vi "Update State Description.vi"(8 "error in (no error)":errorcluster, 9 "description":string, 10 "State":string, 11 "Channel Ref in":T1 format="%.0x") -> (0 "error out":errorcluster, 3 "Channel Ref out":T1=18446744073709551615 format="%.0x")   [LabVIEW 2017, in "Switch Scripting.lvlib"]
uses:
  Switch Scripting.lvlib
  <vilib>/NI Veristand/Custom Device API/Custom Device Item Ref.ctl
  <vilib>/NI VeriStand/Custom Device API/Custom Device API.lvlib
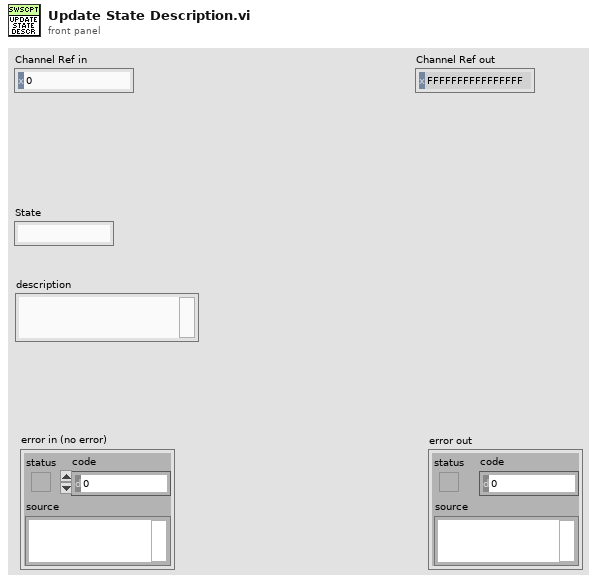
[diagram p1: front panel]
types:
  T1 = typedef "Custom Device API.lvlib/Custom Device Item Ref.ctl" = u64
  T2 = typedef "Switch Scripting.lvlib/Routing State.ctl" = cluster{"name":string, "description":string, "value":i32, "connection list":T3[]}
  T3 = typedef "Switch Scripting.lvlib/Connection.ctl" = cluster{"source":string, "destination":string}
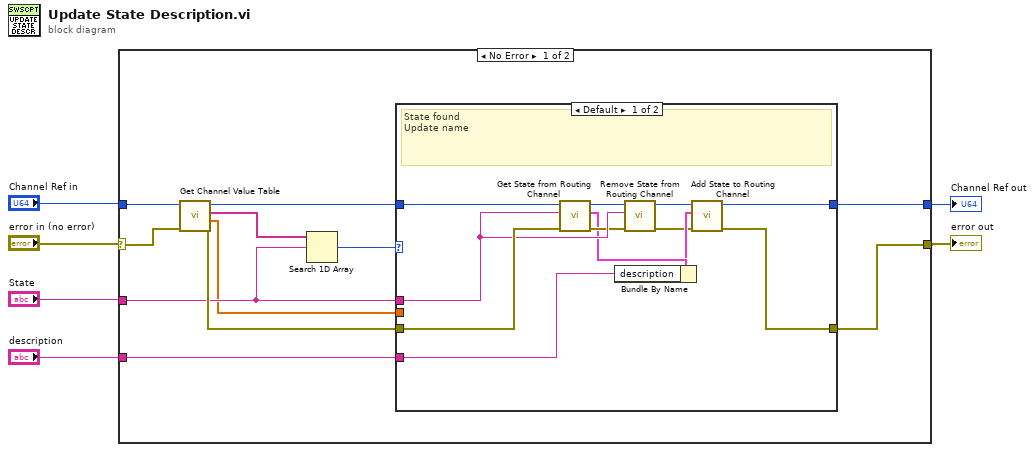
[diagram p0: block diagram]
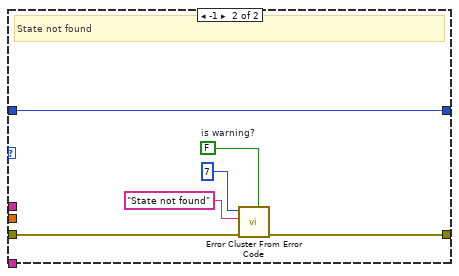
[diagram p2: hidden frame]
diagram:
  n1 = case shown="No Error" "error in (no error)" {
    selector: "error in (no error)" -> [w16 w37]
    tunnel: [w12 w37] -> w2
    tunnel: "Channel Ref in" -> [w17 w36]
    tunnel: [w13 w36] -> w1
    tunnel: "State" -> [w10 _]
    tunnel: "description" -> [w8 _]
    frame No Error {
      n2 = call "Get Channel Value Table.vi"("error in (no error)"=w16, "Channel Ref in"=w17) -> ("error out"=w14:errorcluster, "Values"=w9:dbl[], "States"=w11:string[], "Channel Ref out"=w15:T1)  [unwired: 6 in]
      n3 = Search 1D Array(1D array=w11, element=w10) -> (index of element=w7:i32)  [unwired: 1 in]
      n4 = case shown="Default" w7 {
        tunnel: w15 -> [w29 w30]
        tunnel: w14 -> [w28 w32]
        tunnel: w9 -> [_ _]
        tunnel: [w25 w30] -> w13
        tunnel: [w26 w31] -> w12
        tunnel: w8 -> [w18 _]
        tunnel: w10 -> [w27 _]
        frame Default {
          # "State found\nUpdate name"
          n5 = call "Get State from Routing Channel.vi"("error in (no error)"=w28, "State"=w27, "Channel Ref in"=w29) -> ("error out"=w23:errorcluster, "Routing State"=w22:T2, "Channel Ref out"=w24:T1)  [unwired: 6 in]
          n6 = Bundle By Name(cluster=w22, "description"=w18) -> (w21:T2)
          n7 = call "Remove State from Routing Channel.vi"("error in (no error)"=w23, "State"=w27, "Channel Ref in"=w24) -> ("error out"=w19:errorcluster, "Channel Ref out"=w20:T1)  [unwired: 7 in]
          n8 = call "Add State to Routing Channel.vi"("error in (no error)"=w19, "Routing State"=w21, "Channel Ref in"=w20) -> ("error out"=w26:errorcluster, "Channel Ref out"=w25:T1)  [unwired: 7 in]
        }
        frame -1 {
          w34 = FALSE  # is warning?
          # "State not found"
          n9 = call <vilib>:"Error Cluster From Error Code.vi"("is warning? (False)"=w34, "error in (no error)"=w32, "error message (\"\")"="State not found" ("error message (\"\")"), "error code (0)"=7) -> ("error out"=w31:errorcluster)  [unwired: 5 in]
        }
      }
    }
    frame Error {
    }
  }
  "Channel Ref out" <- w1
  "error out" <- w2
